vi "Find Ref Data Placeholder.vi"(10 "error in (no error)":errorcluster, 11 "VI Refnum":refnum<vi>) -> (2 "error out":errorcluster, 3 "Ref Data Placeholder":refnum<vi>)   [LabVIEW 2018, in "LVClassByRef.lvlib"]
uses:
  <resource>/Framework/Providers/LVClassByRef/LVClassByRef.lvlib
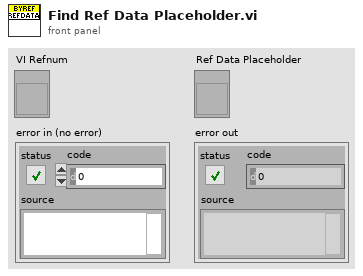
[diagram p1: front panel]
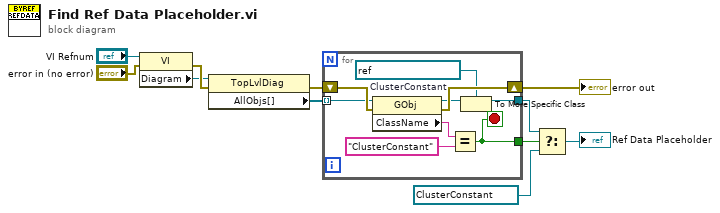
[diagram p0: block diagram]
diagram:
  n1 = property class="VI"(reference="VI Refnum", error in="error in (no error)") -> (error out=w11:errorcluster, "Diagram"=w9:refnum<vi>)  [unwired: 1 out]
  n2 = property class="TopLvlDiag"(reference=w9, error in=w11) -> (error out=w6:errorcluster, "AllObjs[]"=w7:refnum<vi>[])  [unwired: 1 out]
  n3 = for {
    tunnel: w7 -> [w14] mode=indexing
    shift-right: [w18] -> w1
    shift-left: w6 -> [w17]
    tunnel: [w13] -> w5
    tunnel: [w15] -> w4
    stop <- w15 stop-if-true
    w12 = refnum<vi> refnum  # ClusterConstant
    n4 = property class="GObj"(reference=w14, error in=w17) -> (reference out=w16:refnum<vi>, error out=w18:errorcluster, "ClassName"=w20:string)
    n5 = Equal?(x=w20, y="ClusterConstant") -> (x = y?=w15:bool)
    n6 = To More Specific Class(target class=w12, reference=w16) -> (specific class reference=w13:refnum<vi>)  [unwired: 1 in, 1 out]
  }
  "error out" <- w1
  n7 = Select(t=w5, s=w4, f=refnum<vi> refnum) -> (s? t:f=→"Ref Data Placeholder":refnum<vi>)
